vi "Get Control Column Ordering - Minimal.vi"(8 "error in (no error)":errorcluster {"code" format="Error %.0f"}, 11 "VIDoc Printer - Confluence In":refnum<class "VIDoc Printer - Confluence.lvclass">) -> (0 "error out":errorcluster {"code" format="Error %.0f"}, 2 "Minimal":T1[](array[typedef]), 3 "VIDoc Printer - Confluence Out":refnum<class "VIDoc Printer - Confluence.lvclass">)   [LabVIEW 2023, in "VIDoc Printer - Confluence.lvlib" / "VIDoc Printer - Confluence.lvclass"]
uses:
  VIDoc Printer - Confluence.lvclass
  Settings/Confluence Printer Settings/Control Info Column.ctl
  VIDoc Printer - Confluence.lvclass/VIDoc Printer - Confluence.ctl
  Settings/Confluence Printer Settings/VIDoc Settings - Confluence.lvclass
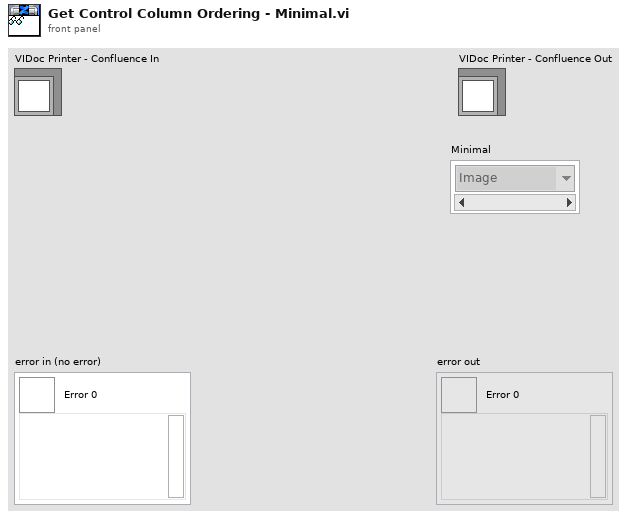
[diagram p1: front panel]
types:
  T1 = typedef "VIDoc Printer - Confluence.lvlib/VIDoc Settings - Confluence.lvclass/Control Info Column.ctl" = enum16{"Image", "Name", "Description", "Caption", "Tip Strip", "Data Type", "Key Toggle"}
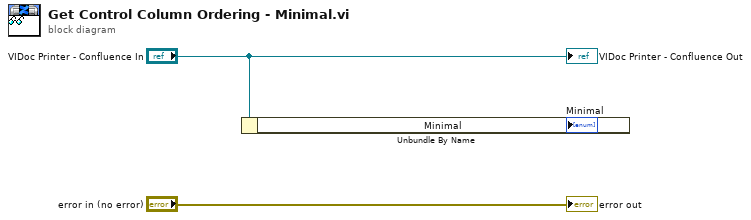
[diagram p0: block diagram]
diagram:
  n1 = Unbundle By Name("VIDoc Printer - Confluence In") -> ("Minimal"=→"Minimal":T1[])
  "error out" <- "error in (no error)"
  "VIDoc Printer - Confluence Out" <- "VIDoc Printer - Confluence In"
